vi "Dictionary Clear__ogtk.vi"(8 "error in (no error)":errorcluster, 11 "dictionary":T1) -> (0 "error out":errorcluster, 3 "dictionary out":T1)   [LabVIEW 2011]
doc: "Clears (Empties) the dictionary."
uses:
  Dictionary Object RefNum__ogtk.ctl
  Dictionary Object RefNum - Enum__ogtk.ctl
panel:
  # "Dictionary Clear.vi\n\nClears (Empties) the dictionary.\n\nPlease visit http://www.OpenG.org to learn about the\nOpen Source LabVIEW software movement.\n\nNOTICE -- YOU MUST LEAVE THIS NOTICE IN PLACE.  PER THE TERMS OF THE LICENSE BELOW, YOU MAY SUBLICENSE THIS SOFTWARE \nIN ANY WAY THAT DOES NOT CONFLICT WITH THIS LICENSE.\n\n### BSD License (http://www.opensource.org/licenses/bsd-license.php) Begin ###\n \nCopyright (c) 2005, Jim Kring <jim@jimkring.com>\n\nAll rights reserved.\n\nRedistribution and use in source and binary forms, with or without modification, are permitted provided that the following conditions are met:\n\n    * Redistributions of source code must retain the above copyright notice, this list of conditions and the following disclaimer.\n    * Redistributions in binary form must reproduce the above copyright notice, this list of conditions and the following disclaimer in the \n       documentation and/or other materials provided with the distribution.\n    * Neither the name of SciWare, James Kring, Inc., nor the names of its contributors may be used to endorse or promote products derived \n       from this software without specific prior written permission.\n\nTHIS SOFTWARE IS PROVIDED BY THE COPYRIGHT HOLDERS AND CONTRIBUTORS \"AS IS\" AND ANY EXPRESS OR IMPLIED WARRANTIES, \nINCLUDING, BUT NOT LIMITED TO, THE IMPLIED WARRANTIES OF MERCHANTABILITY AND FITNESS FOR A PARTICULAR PURPOSE ARE \nDISCLAIMED. IN NO EVENT SHALL THE COPYRIGHT OWNER OR CONTRIBUTORS BE LIABLE FOR ANY DIRECT, INDIRECT, INCIDENTAL,\n SPECIAL, EXEMPLARY, OR CONSEQUENTIAL DAMAGES (INCLUDING, BUT NOT LIMITED TO, PROCUREMENT OF SUBSTITUTE GOODS OR \nSERVICES; LOSS OF USE, DATA, OR PROFITS; OR BUSINESS INTERRUPTION) HOWEVER CAUSED AND ON ANY THEORY OF LIABILITY, \nWHETHER IN CONTRACT, STRICT LIABILITY, OR TORT (INCLUDING NEGLIGENCE OR OTHERWISE) ARISING IN ANY WAY OUT OF THE USE \nOF THIS SOFTWARE, EVEN IF ADVISED OF THE POSSIBILITY OF SUCH DAMAGE.\n\n### BSD License End ###"
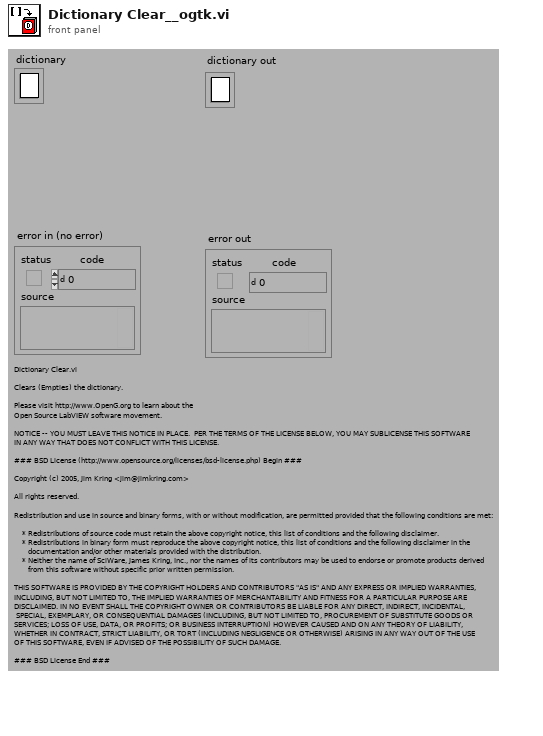
[diagram p1: front panel]
types:
  T1 = typedef "Dictionary Object RefNum__ogtk.ctl" = refnum<k1>
  T2 = typedef "Dictionary Data__ogtk.ctl" = cluster{"keys":variant[], "values":variant[]}
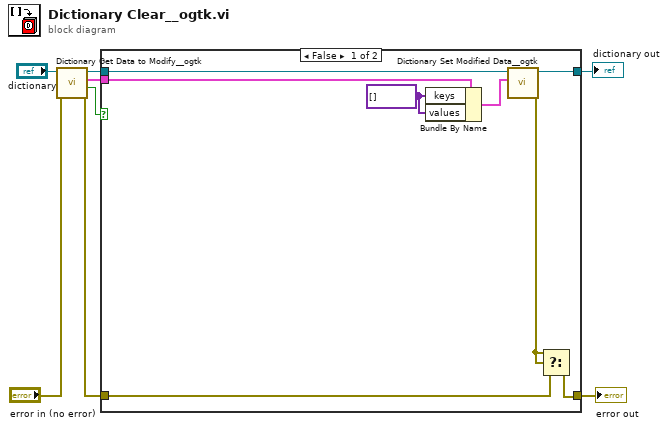
[diagram p0: block diagram]
diagram:
  n1 = call "Dictionary Get Data to Modify__ogtk.vi"("error in (no error)"="error in (no error)", "Object RefNum"="dictionary") -> ("error out"=w5:errorcluster, "timed out"=w4:bool, "Data out"=w6:T2, "Dup Object RefNum"=w1:T1)  [unwired: 6 in]
  n2 = case shown="False" w4 {
    tunnel: w6 -> [w10 _]
    tunnel: w5 -> [w12 w18]
    tunnel: [w11 w18] -> w7
    tunnel: [w15 w17] -> w2
    tunnel: w1 -> [w14 w17]
    frame False {
      w9 = variant[] [] ("keys")
      n3 = Bundle By Name(cluster=w10, "keys"=w9, "values"=w9) -> (w16:T2)
      n4 = call "Dictionary Set Modified Data__ogtk.vi"("Data in"=w16, "Object RefNum"=w14) -> ("error out"=w13:errorcluster, "dup Object RefNum"=w15:T1)  [unwired: 8 in]
      n5 = Select(t=w13, s=w13, f=w12) -> (s? t:f=w11:errorcluster)
    }
    frame True {
      # "Error or timed out"
    }
  }
  "error out" <- w7
  "dictionary out" <- w2
